vi "Configure 2Wire Resistance.vi"(0 "VISA resource name":refnum<visa-resource-name>, 1 "Aperture Seconds":dbl, 5 "Auto Range? (T: Auto)":bool, 7 "Manual Range":dbl=1000.0, 9 "Set Aperture or NPLC":bool=TRUE, 11 "error in (no error)":errorcluster, 12 "NPLC":dbl=1.0) -> (4 "VISA resource name out":refnum<visa-resource-name>, 15 "error out":errorcluster)   [LabVIEW 2021, in "Keithley DMM7510.lvlib"]
doc: "This VI configures the 2 wire Resistance."
uses:
  Keithley DMM7510.lvlib
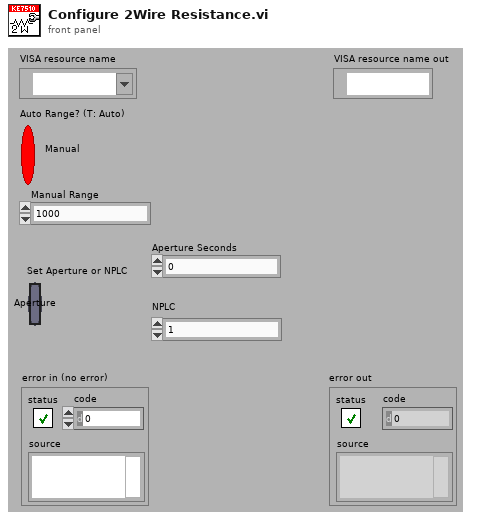
[diagram p1: front panel]
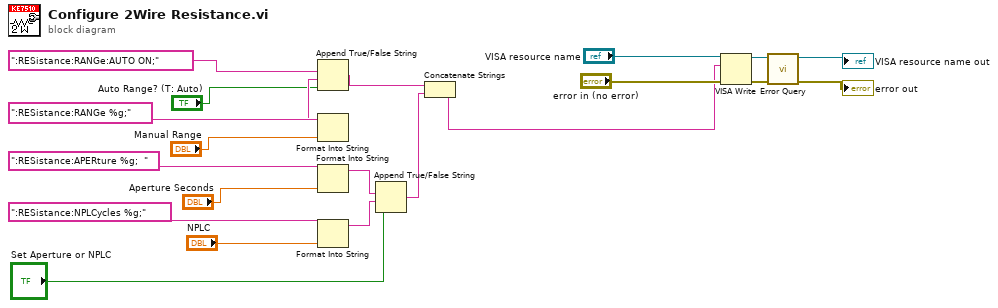
[diagram p0: block diagram]
diagram:
  n1 = Format Into String(format string=":RESistance:RANGe %g;", "Manual Range") -> (resulting string=w13:string)  [unwired: 2 in, 1 out]
  n2 = Append True/False String(1:"Auto Range? (T: Auto)", 2:w13, 3:":RESistance:RANGe:AUTO ON;") -> (0:w10:string)  [unwired: 1 in]
  n3 = Format Into String(format string=":RESistance:APERture %g;  ", "Aperture Seconds") -> (resulting string=w4:string)  [unwired: 2 in, 1 out]
  n4 = Format Into String(format string=":RESistance:NPLCycles %g;", "NPLC") -> (resulting string=w3:string)  [unwired: 2 in, 1 out]
  n5 = Append True/False String(1:"Set Aperture or NPLC", 2:w3, 3:w4) -> (0:w1:string)  [unwired: 1 in]
  n6 = Concatenate Strings(w10, w1) -> (w9:string)
  n7 = VISA Write(VISA resource name="VISA resource name", write buffer=w9, error in (no error)="error in (no error)") -> (VISA resource name out=w21:refnum<visa-resource-name>, error out=w20:errorcluster)  [unwired: 1 out]
  n8 = call "Error Query.vi"("error in (no error)"=w20, "VISA resource name"=w21) -> ("error out"=→"error out":errorcluster, "VISA resource name out"=→"VISA resource name out":refnum<visa-resource-name>)  [unwired: 6 in, 2 out]
